vi "VIRefProbe.vi"(11 "VI Refnum":refnum<vi>) -> (2 "Value String":string, 3 "Stop?":bool)   [LabVIEW 2017]
doc: "Displays the VI name, the VI path, and the hex value of the reference. You can use this probe to set a breakpoint if the value is an invalid refnum."
uses:
  <vilib>/Utility/error.llb/DialogTypeEnum.ctl
panel:
  in  "vi application instance":string="Application instance"
  in  "error source":string="VI Refnum Probe"
  in  "vi path":string="VI path"
  in  "vi name":string="VI name"
  out "Display string":string
  in  "Pause if Not a Refnum":bool
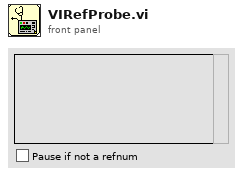
[diagram p1: front panel]
types:
  T1 = typedef "DialogTypeEnum.ctl" = enum16{"no dialog", "OK message", "continue or stop message", "auto error handling dialog", "OK message + warnings", "continue/stop + warnings"}
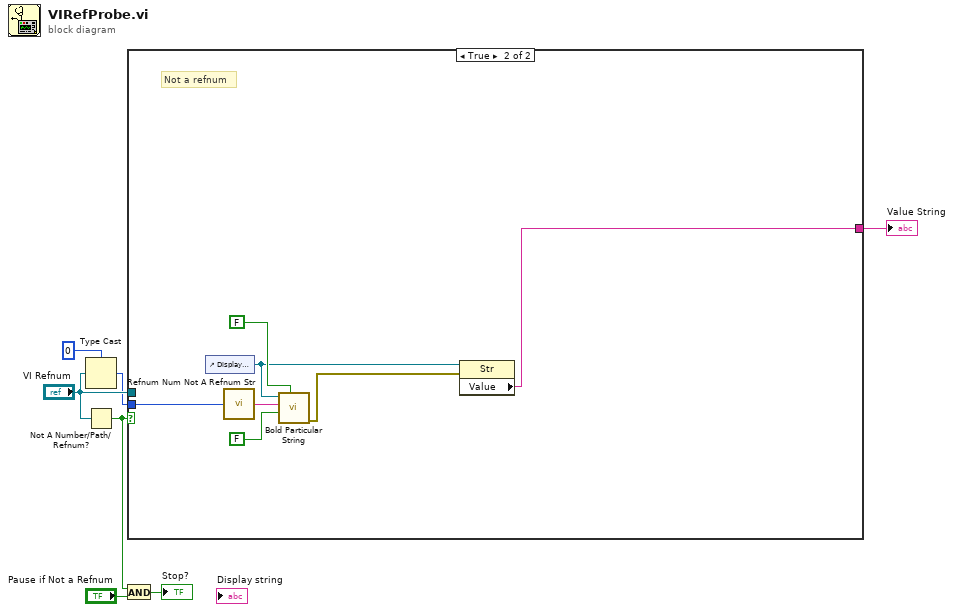
[diagram p0: block diagram]
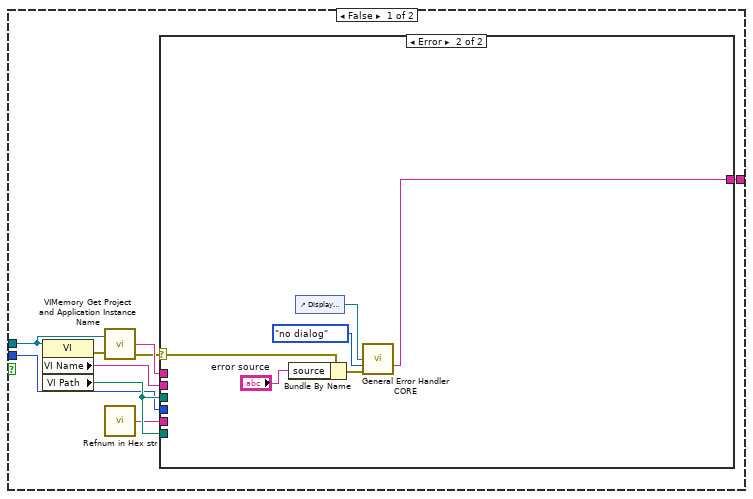
[diagram p2: hidden frame]
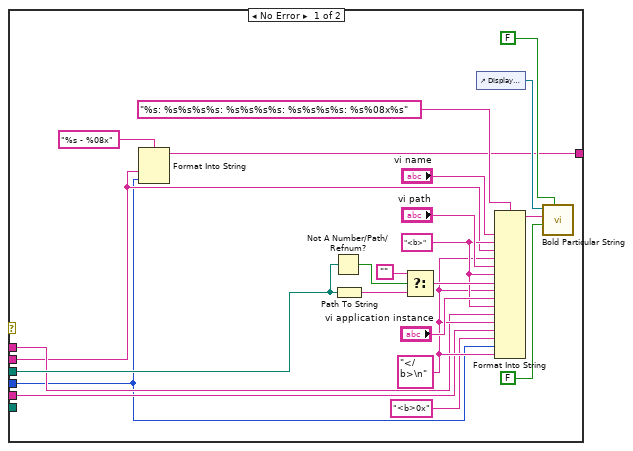
[diagram p3: hidden frame]
diagram:
  n1 = Type Cast(type=u32 0, x="VI Refnum") -> (*(type *) &x=w2:u32)
  n2 = Not A Number/Path/Refnum?(number/path/refnum="VI Refnum") -> (NaN/Path/Refnum?=w5:bool)
  n3 = And(x=w5, y="Pause if Not a Refnum") -> (x .and. y?=→"Stop?":bool)
  n4 = case shown="True" w5 {
    tunnel: "VI Refnum" -> [w11 _]
    tunnel: w2 -> [w14 w49]
    tunnel: [w8 w46] -> w1
    frame False {
      n5 = property class="VI"(reference=w11) -> (error out=w10:errorcluster, "VI Name"=w16:string, "VI Path"=w15:path)  [unwired: 1 in, 1 out]
      n6 = call <vilib>:"VIMemory Get Project and Application Instance Name.vi"("vi reference"=w11, "error in (no error)"=w10) -> ("Project and Application Instance Name"=w12:string, "error out"=w9:errorcluster)  [unwired: 1 out]
      n7 = call <vilib>:"Refnum in Hex str.vi"() -> ("refnum in hex"=w13:string)
      n8 = case shown="Error" w9 {
        selector: w9 -> [_ w41]
        tunnel: w14 -> [w18 _]
        tunnel: w13 -> [w22 _]
        tunnel: w15 -> [_ _]
        tunnel: w16 -> [w19 _]
        tunnel: w15 -> [w33 _]
        tunnel: w12 -> [w23 _]
        tunnel: [w17 w39] -> w8
        frame No Error {
          w24 = "</b>\n"
          w25 = "<b>"
          n9 = Format Into String(format string="%s - %08x", w19, w18) -> (resulting string=w17:string)  [unwired: 2 in, 1 out]
          n10 = Not A Number/Path/Refnum?(number/path/refnum=w33) -> (NaN/Path/Refnum?=w36:bool)
          n11 = Path To String(path=w33) -> (string=w35:string)
          n12 = Select(t="", s=w36, f=w35) -> (s? t:f=w30:string)
          n13 = control-ref of="Display string"() -> (w38:refnum<vi>)
          n14 = Format Into String(format string="%s: %s%s%s%s: %s%s%s%s: %s%s%s%s: %s%08x%s", "vi name", w25, w19, w24, "vi path", w25, w30, w24, "vi application instance", w25, w23, w24, w22, "<b>0x", w18, w24) -> (resulting string=w31:string)  [unwired: 2 in, 1 out]
          n15 = call <vilib>:"Bold Particular String.vi"("Always Refresh? (TRUE)"=FALSE ("Always Refresh? (FALSE)"), "resize string? (TRUE)"=FALSE ("resize string?"), "text to display"=w31, "string refnum"=w38) -> ()  [unwired: 1 in, 7 out]
        }
        frame Error {
          n16 = Bundle By Name(cluster=w41, "source"="error source") -> (w43:errorcluster)
          n17 = control-ref of="Display string"() -> (w40:refnum<vi>)
          n18 = call <vilib>:"General Error Handler CORE.vi"("String to Format (not a refnum)"=w40, "type of dialog (OK msg:1)"=DialogTypeEnum."no dialog", "error in (no error)"=w43) -> ("message"=w39:string)  [unwired: 12 out]
        }
      }
    }
    frame True {
      # "Not a refnum"
      n19 = control-ref of="Display string"() -> (w47:refnum<vi>)
      n20 = call <vilib>:"Refnum Num Not A Refnum Str.vi"("Numeric"=w49) -> ("text to display"=w48:string)
      n21 = call <vilib>:"Bold Particular String.vi"("Always Refresh? (TRUE)"=FALSE ("Always Refresh? (FALSE)"), "resize string? (TRUE)"=FALSE, "text to display"=w48, "string refnum"=w47) -> ("error out"=w45:errorcluster)  [unwired: 1 in, 6 out]
      n22 = property class="Str"(reference=w47, error in=w45) -> ("Value"=w46:string)  [unwired: 2 out]
    }
  }
  "Value String" <- w1
